vi "Populate Attribute Details.vi"(8 "error in":errorcluster, 9 "Sub-Index":string, 10 "Index":string, 11 "UI Actor in":refnum<class "UI Actor.lvclass">) -> (0 "error out":errorcluster, 3 "UI Actor out":refnum<class "UI Actor.lvclass">)   [LabVIEW 2024, in "UI Actor.lvlib" / "UI Actor.lvclass"]
uses:
  UI Actor.lvclass
  UI Actor.lvclass/UI Actor.ctl
  Core/OD Entry/OD Entry.lvclass
  Electronic Datasheet/Electronic Datasheet.lvclass
  Core/Object Type.ctl
  Core/Electronic Datasheet.lvlib
  Core/Access SDO.ctl
  Core/Access PDO.ctl
  Core/Access SRDO.ctl
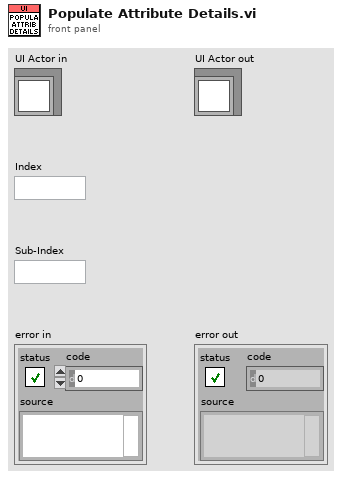
[diagram p1: front panel]
types:
  T1 = map{path, refnum<class "Electronic Datasheet.lvclass">}
  T2 = typedef "Electronic Datasheet.lvlib/Object Type.ctl" = u8
  T3 = typedef "Electronic Datasheet.lvlib/Access SDO.ctl" = enum16{"read only", "write only", "read/write", "read/write on process input", "read/write on process output", "constant value", "no", "UNKNOWN"}
  T4 = typedef "Electronic Datasheet.lvlib/Access PDO.ctl" = enum16{"no", "t", "r", "tr"}
  T5 = typedef "Electronic Datasheet.lvlib/Access SRDO.ctl" = enum16{"no", "tx", "rx", "trx"}
  T6 = cluster{"ParameterName":string, "Description":string, "ObjectType":T2, "DataType":u16, "DefaultValue":string, "Denotation":string, "HighLimit":string, "LowLimit":string, "Access SDO":T3, "Access PDO":T4, "Access SRDO":T5, "Actual Value":string}
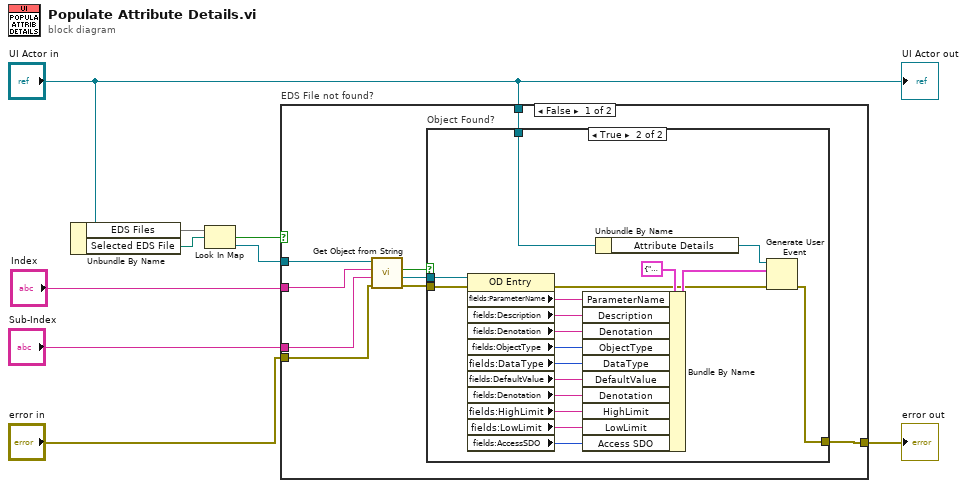
[diagram p0: block diagram]
diagram:
  n1 = Unbundle By Name("UI Actor in") -> ("EDS Files"=w9:T1, "Selected EDS File"=w8:path)
  n2 = Look In Map(map=w9, key=w8) -> (key not found?=w2:bool, value=w7:refnum<class "Electronic Datasheet.lvclass">)  [unwired: 1 in]
  n3 = case "EDS File not found?" shown="False" w2 {
    tunnel: w7 -> [w16 _]
    tunnel: "error in" -> [w12 w38]
    tunnel: [w14 w38] -> w5
    tunnel: "UI Actor in" -> [w15 _]
    tunnel: "Index" -> [w10 _]
    tunnel: "Sub-Index" -> [w13 _]
    frame False {
      n4 = call "Get Object from String.vi"("error in"=w12, "Sub-Index"=w13, "Index"=w10, "reference in"=w16) -> ("error out"=w11:errorcluster, "OD Entry"=w18:refnum<class "OD Entry.lvclass">, "Found?"=w17:bool)  [unwired: 4 in, 1 out]
      n5 = case "Object Found?" shown="True" w17 {
        tunnel: w11 -> [w19 w31]
        tunnel: w18 -> [_ w32]
        tunnel: w15 -> [_ w37]
        tunnel: [w19 w33] -> w14
        frame False {
        }
        frame True {
          n6 = property class="OD Entry"(reference=w32, error in=w31) -> (error out=w30:errorcluster, "fields:ParameterName"=w29:string, "fields:Description"=w28:string, "fields:Denotation"=w27:string, "fields:ObjectType"=w26:T2, "fields:DataType"=w25:u16, "fields:DefaultValue"=w24:string, "fields:Denotation"=w23:string, "fields:HighLimit"=w22:string, "fields:LowLimit"=w21:string, "fields:AccessSDO"=w20:T3)  [unwired: 1 out]
          n7 = Bundle By Name(cluster=T6 {"ParameterName"="", "Description"="", "ObjectType"=0, "DataType"=0, "DefaultValue"="", "Denotation"="", "HighLimit"="", "LowLimit"="", "Access SDO"=enum."read only", "Access PDO"=enum."no", "Access SRDO"=enum."no", "Actual Value"=""} ("event data"), "ParameterName"=w29, "Description"=w28, "Denotation"=w27, "ObjectType"=w26, "DataType"=w25, "DefaultValue"=w24, "Denotation"=w23, "HighLimit"=w22, "LowLimit"=w21, "Access SDO"=w20) -> (w34:T6)
          n8 = Unbundle By Name(w37) -> ("Attribute Details"=w36:refnum<user-event>)
          n9 = Generate User Event(user event=w36, event data cluster=w34, error in=w30) -> (error out=w33:errorcluster)  [unwired: 1 in, 1 out]
        }
      }
    }
    frame True {
    }
  }
  "error out" <- w5
  "UI Actor out" <- "UI Actor in"
